vi "ISX3_Parse_FrequencyPoint.vi"(0 "Array":u8[](array[numeric])) -> (1 "Frequency [Hz]":sgl, 2 "Precision":sgl, 3 "Amplitude [V]":sgl)   [LabVIEW 2012, in "Sciospec ISX3 Impedance Analyzer.lvlib"]
uses:
  Sciospec ISX3 Impedance Analyzer.lvlib
panel:
  # "This VI parses a data frame that contains a setup row."
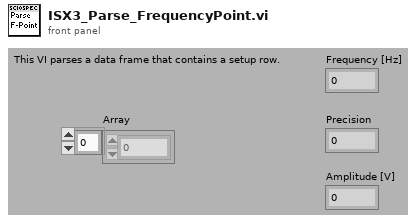
[diagram p1: front panel]
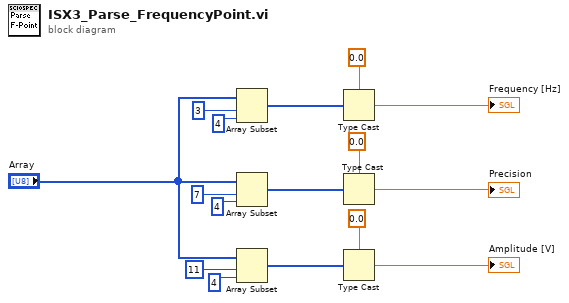
[diagram p0: block diagram]
diagram:
  n1 = Array Subset(array="Array", index=3 ("Index"), length=4 ("Länge")) -> (w15:u8[])
  n2 = Array Subset(array="Array", index=7 ("Index"), length=4 ("Länge")) -> (w10:u8[])
  n3 = Array Subset(array="Array", index=11 ("Index"), length=4 ("Länge")) -> (w2:u8[])
  n4 = Type Cast(type=sgl 0.0, x=w15) -> (*(type *) &x=→"Frequency [Hz]":sgl)
  n5 = Type Cast(type=sgl 0.0, x=w10) -> (*(type *) &x=→"Precision":sgl)
  n6 = Type Cast(type=sgl 0.0, x=w2) -> (*(type *) &x=→"Amplitude [V]":sgl)
